vi "Database.vi"(4 "Maximum Row":i32, 5 "Enum":enum16{"ID Delete", "Time Delete"}(ring), 6 "Delete row?":bool, 7 "Data":variant, 8 "Error in":errorcluster, 9 "Auto Increment ID?":bool, 10 "Table":string, 11 "Connection":string) -> (0 "Error out":errorcluster)   [LabVIEW 2019, in "database.lvlib"]
uses:
  database.lvlib
  <vilib>/addons/database/Connection.llb/DB Tools Open Connec (String).vi
  <vilib>/addons/database/_DB Variant To Data/Database Variant To Data.xnode
  <vilib>/addons/database/NI_Database_API.lvlib
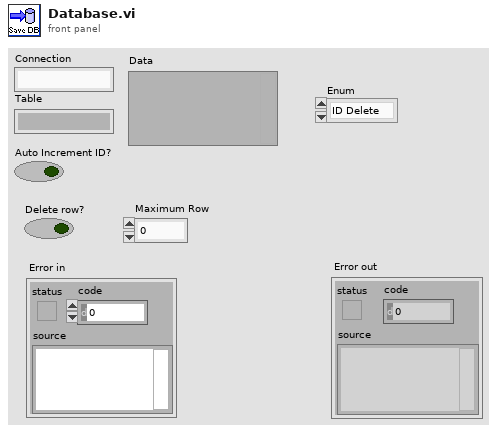
[diagram p1: front panel]
types:
  T1 = typedef "NI_Database_API.lvlib/Conn ObjectReference.ctl" = refnum<k1>
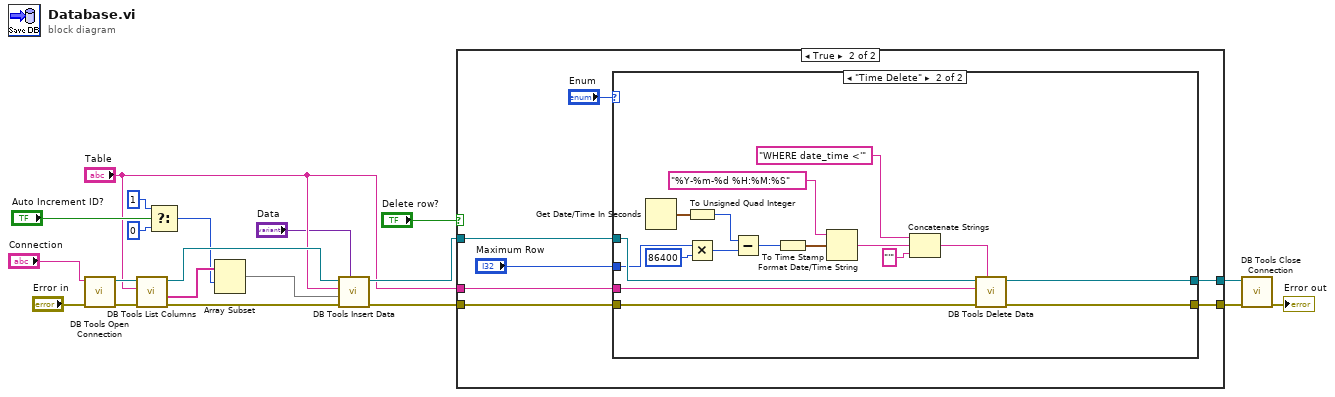
[diagram p0: block diagram]
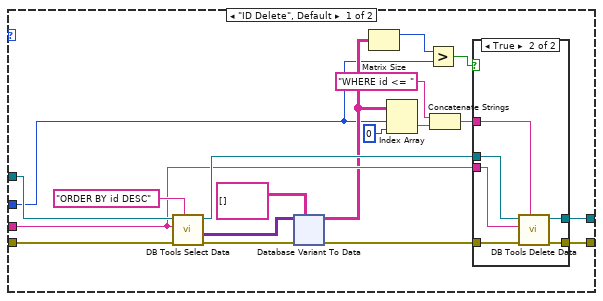
[diagram p3: hidden frame]
diagram:
  n1 = call-poly <vilib>:"DB Tools Open Connection.vi"("error in (no error)"="Error in", "connection information"="Connection") -> ("error out"=w18:errorcluster, "connection reference"=w20:T1)  [unwired: 6 in]
  n2 = call <vilib>:"DB Tools List Columns.vi"("error in (no error)"=w18, "table"="Table", "connection reference"=w20) -> ("error out"=w17:errorcluster, "columns"=w11:string[], "connection reference out"=w19:T1)  [unwired: 1 in, 1 out]
  n3 = Select(t=1 ("index"), s="Auto Increment ID?", f=0) -> (s? t:f=w8:i32)
  n4 = Array Subset(array=w11, index=w8) -> (w7:string[])  [unwired: 1 in]
  n5 = call <vilib>:"DB Tools Insert Data.vi"("data"="Data", "error in (no error)"=w17, "columns"=w7, "table"="Table", "connection reference"=w19) -> ("error out"=w16:errorcluster, "connection reference out"=w15:T1)  [unwired: 5 in]
  n6 = case shown="True" "Delete row?" {
    tunnel: w16 -> [w21 w29]
    tunnel: w15 -> [w22 w28]
    tunnel: "Table" -> [_ w27]
    tunnel: [w21 w26] -> w2
    tunnel: [w22 w25] -> w1
    frame False {
    }
    frame True {
      n7 = case shown="\"Time Delete\"" "Enum" {
        tunnel: w29 -> [w47 w117]
        tunnel: w28 -> [w48 w116]
        tunnel: w27 -> [w36 w115]
        tunnel: [w39 w114] -> w26
        tunnel: [w38 w113] -> w25
        tunnel: "Maximum Row" -> [w34 w101]
        frame "ID Delete", Default {
          n8 = call <vilib>:"DB Tools Select Data.vi"("condition"="ORDER BY id DESC", "error in (no error)"=w47, "table"=w36, "connection reference"=w48) -> ("error out"=w45:errorcluster, "data"=w46:variant[][], "connection reference out"=w37:T1)  [unwired: 2 in]
          n9 = xnode "Database Variant To Data"("database variant"=w46, "error in (no error)"=w45, "type"=string[][] []) -> ("data"=w35:string[][], "error out"=w40:errorcluster)
          n10 = Matrix Size(0:w35) -> (1:w42:i32)  [unwired: 1 out]
          n11 = Index Array(array=w35, index (row)=w34, index (col)=0 ("disabled index (col)")) -> (element=w32:string)
          n12 = Greater?(x=w42, y=w34) -> (0:w41:bool)
          n13 = Concatenate Strings("WHERE id <= " ("string"), w32) -> (w30:string)
          n14 = case shown="True" w41 {
            tunnel: w40 -> [w50 w56]
            tunnel: [w50 w55] -> w39
            tunnel: [w49 w54] -> w38
            tunnel: w37 -> [w49 w53]
            tunnel: w36 -> [_ w52]
            tunnel: w30 -> [_ w51]
            frame False {
            }
            frame True {
              n15 = call <vilib>:"DB Tools Delete Data.vi"("condition"=w51, "error in (no error)"=w56, "table"=w52, "connection reference"=w53) -> ("error out"=w55:errorcluster, "connection reference out"=w54:T1)  [unwired: 6 in]
            }
          }
        }
        frame "Time Delete" {
          n16 = Get Date/Time In Seconds() -> (seconds since 1Jan1904=w108:timestamp)
          n17 = To Unsigned Quad Integer(1:w108) -> (0:w111:u64)
          n18 = Multiply(x=w101, y=u64 86400) -> (x*y=w110:u64)
          n19 = Subtract(x=w111, y=w110) -> (x-y=w112:u64)
          n20 = To Time Stamp(1:w112) -> (0:w107:timestamp)
          n21 = Format Date/Time String(time format string (%c)="%Y-%m-%d %H:%M:%S", seconds (now)=w107) -> (date/time string=w109:string)  [unwired: 1 in]
          n22 = Concatenate Strings("WHERE date_time <'" ("string"), w109, "'" ("string")) -> (w102:string)
          n23 = call <vilib>:"DB Tools Delete Data.vi"("condition"=w102, "error in (no error)"=w117, "table"=w115, "connection reference"=w116) -> ("error out"=w114:errorcluster, "connection reference out"=w113:T1)  [unwired: 6 in]
        }
      }
    }
  }
  n24 = call <vilib>:"DB Tools Close Connection.vi"("error in (no error)"=w2, "connection reference"=w1) -> ("error out"=→"Error out":errorcluster)  [unwired: 5 in]
